vi "SEQPool.vi"(0 "Pool in":refnum<vi>, 1 "SEQ in":refnum<class "Sequence.lvclass">[](array[class])) -> (8 "SEQ out":refnum<class "Sequence.lvclass">[](array[class]))   [LabVIEW 2012, in "StimulCtrls.lvlib"]
uses:
  StimulCtrls.lvlib
  SEQPool.ctl
  UserControl/Cohort_sm.ctl
  UserControl/ElectdTerminal.ctl
  Sequence.lvclass
  Cohort.lvclass
panel:
  in  "Pool":T1
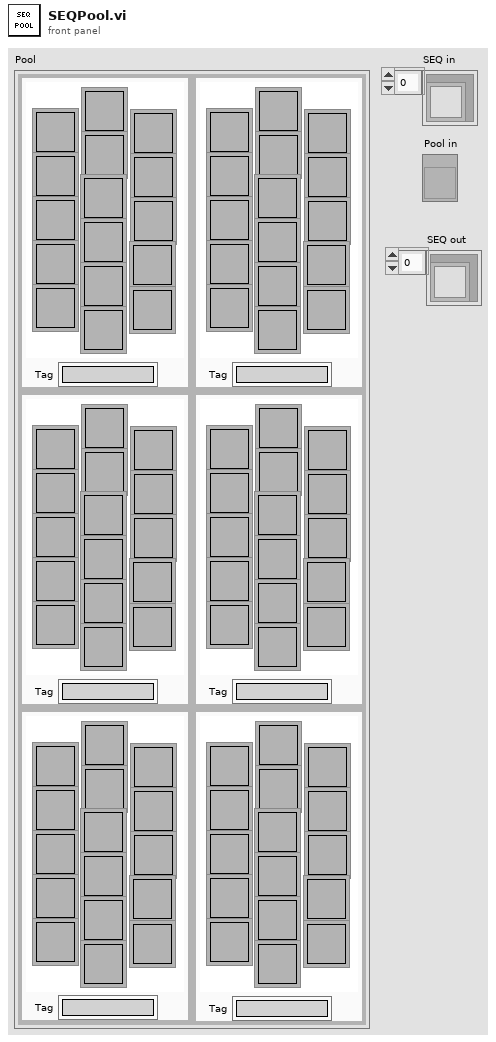
[diagram p1: front panel]
types:
  T1 = typedef "StimulCtrls.lvlib/SEQPool.ctl" = cluster{"Seed 0":T2, "Seed 1":T2, "Seed 2":T2, "Seed 3":T2, "Seed 4":T2, "Seed 5":T2}
  T2 = typedef "StimulCtrls.lvlib/Cohort_sm.ctl" = cluster{"Simplified Panel":cluster{"Ring 0":cluster{"T 0":T3}, "Ring 1":cluster{"T 0":T3}, "Ring 2":cluster{"T 0":T3}, "Ring 3":cluster{"T 0":T3}, "Ring 4":cluster{"T 0":T3}, "Ring 5":cluster{"T 0":T3}, "Ring 6":cluster{"T 0":T3}, "Ring 7":cluster{"T 0":T3}, "Ring 8":cluster{"T 0":T3}, "Ring 9":cluster{"T 0":T3}, "Ring 10":cluster{"T 0":T3}, "Ring 11":cluster{"T 0":T3}, "Ring 12":cluster{"T 0":T3}, "Ring 13":cluster{"T 0":T3}, "Ring 14":cluster{"T 0":T3}, "Ring 15":cluster{"T 0":T3}}, "Tag":string}
  T3 = typedef "StimulCtrls.lvlib/ElectdTerminal.ctl" = u8
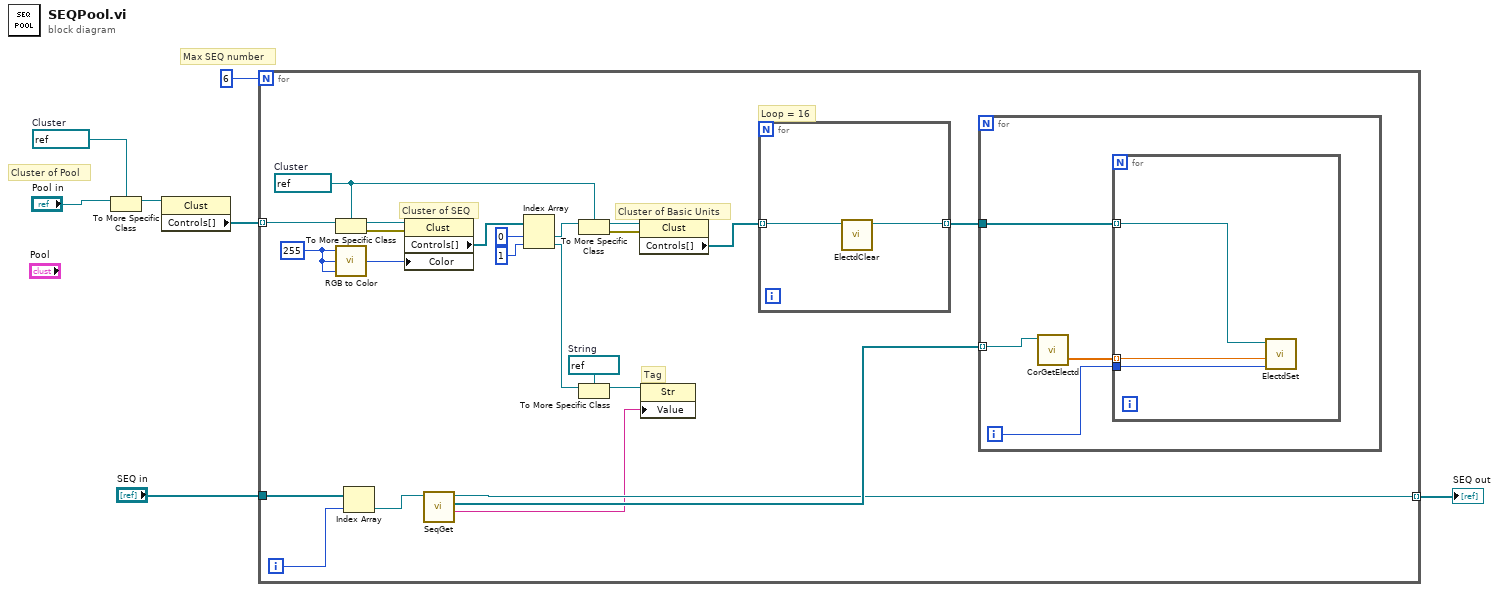
[diagram p0: block diagram]
diagram:
  w3 = refnum<vi> refnum  # Cluster
  # "Cluster of Pool"
  # "Max SEQ number"
  n1 = To More Specific Class(target class=w3, reference="Pool in") -> (specific class reference=w4:refnum<vi>)  [unwired: 1 in, 1 out]
  n2 = property class="Clust"(reference=w4) -> ("Controls[]"=w7:refnum<vi>[])  [unwired: 1 in, 2 out]
  n3 = for {
    N: 6 -> [_]
    tunnel: "SEQ in" -> [w23]
    tunnel: w7 -> [w30] mode=indexing
    tunnel: [w24] -> w6 mode=indexing
    i -> [w22]
    w9 = refnum<vi> refnum  # String
    w20 = u8 255 ("R")
    w15 = refnum<vi> refnum  # Cluster
    # "Tag"
    # "Cluster of Basic Units"
    # "Cluster of SEQ"
    # "Loop = 16"
    n4 = To More Specific Class(target class=w15, reference=w30) -> (specific class reference=w29:refnum<vi>, error out=w28:errorcluster)  [unwired: 1 in]
    n5 = call <vilib>:"RGB to Color.vi"("B"=w20, "G"=w20, "R"=w20) -> ("Color"=w19:u32)
    n6 = Index Array(array=w23, index=w22) -> (element=w21:refnum<class "Sequence.lvclass">)
    n7 = property class="Clust"(reference=w29, error in=w28, "Color"=w19) -> ("Controls[]"=w27:refnum<vi>[])  [unwired: 2 out]
    n8 = call-dynamic "SeqGet.vi"("Sequence in"=w21) -> ("Tag"=w8:string, "Cohorts"=w25:refnum<class "Cohort.lvclass">[], "Sequence out"=w24:refnum<class "Sequence.lvclass">)  [unwired: 7 in, 1 out]
    n9 = Index Array(array=w27, index #1=0 ("index"), index #2=1 ("index")) -> (element #1=w18:refnum<vi>, element #2=w11:refnum<vi>)
    n10 = To More Specific Class(target class=w15, reference=w18) -> (specific class reference=w16:refnum<vi>, error out=w13:errorcluster)  [unwired: 1 in]
    n11 = To More Specific Class(target class=w9, reference=w11) -> (specific class reference=w10:refnum<vi>)  [unwired: 1 in, 1 out]
    n12 = property class="Clust"(reference=w16, error in=w13) -> ("Controls[]"=w14:refnum<vi>[])  [unwired: 2 out]
    n13 = property class="Str"(reference=w10, "Value"=w8) -> ()  [unwired: 1 in, 2 out]
    n14 = for {
      tunnel: w14 -> [w38] mode=indexing
      tunnel: [w39] -> w26 mode=indexing
      n15 = call "ElectdClear.vi"("Electd in"=w38) -> ("Electd out"=w39:refnum<vi>)  [unwired: 10 in]
    }
    n16 = for {
      tunnel: w25 -> [w34] mode=indexing
      tunnel: w26 -> [w32]
      i -> [w31]
      n17 = call-dynamic "CorGetElectd.vi"("Cohort in"=w34) -> ("Amplitude"=w33:sgl[])  [unwired: 6 in, 4 out]
      n18 = for {
        tunnel: w33 -> [w37] mode=indexing
        tunnel: w32 -> [w35] mode=indexing
        tunnel: w31 -> [w36]
        n19 = call "ElectdSet.vi"("Group #"=w36, "Amplitude"=w37, "Electd Panel in"=w35) -> ()  [unwired: 8 in, 1 out]
      }
    }
  }
  "SEQ out" <- w6
